vi "Read Input Registers1.vi"(7 "Unit_ID":T1={"Protocol ID"=0, "Unit ID"=1}, 8 "error in (no error)":errorcluster, 9 "number of input registers":u16, 10 "starting address":u16, 11 "Modbus master in":refnum<class "TCP.lvclass">) -> (0 "error out":errorcluster, 2 "register values":u16[](array[numeric]), 3 "Modbus master out":refnum<class "TCP.lvclass">)   [LabVIEW 2019, in "NI_modbus_upd.lvlib"]
doc: "Reads values from contiguous input registers. The maximum number of input registers this VI can read is 125."
uses:
  NI_modbus_upd.lvlib
  TCP/TCP.lvclass
  Ctl/Unit_ID.ctl
  TCP/TCP.lvclass/TCP.ctl
  Utility/Bytes to U16s1.vi
  Function code mismatch error1.vi
  Error Generator1.vi
  Read ADU Packet Master.vi
  Write ADU Packet Master.vi
  Modbus Data Unit (PDU)/Construct PDU1.vi
  Modbus Data Unit (PDU)/Unflatten to PDU1.vi
  TCP/Protocol Read.vi
  TCP/Protocol Write.vi
  <vilib>/Utility/error.llb/Error Cluster From Error Code.vi
  Modbus Data Unit (PDU)/Deconstruct PDU1.vi
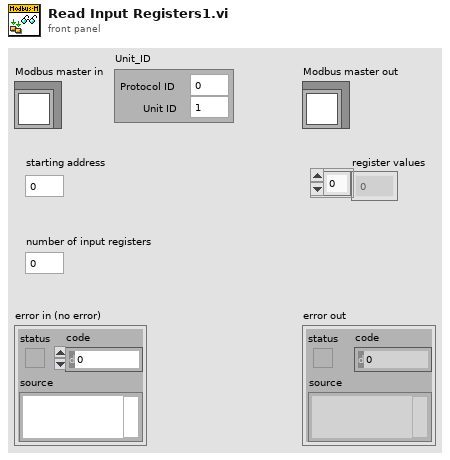
[diagram p1: front panel]
types:
  T1 = typedef "NI_modbus_upd.lvlib/Unit_ID.ctl" = cluster{"Protocol ID":u16, "Unit ID":u8}
  T2 = typedef "NI_modbus_upd.lvlib/MB Modbus Data Unit.ctl" = cluster{"function":T3, "Data":u8[]}
  T3 = typedef "NI_modbus_upd.lvlib/Function.ctl" = u8
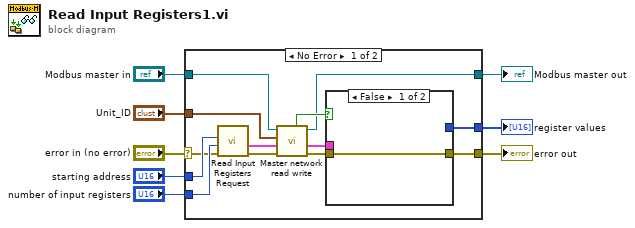
[diagram p0: block diagram]
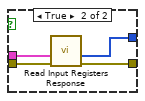
[diagram p2: hidden frame]
diagram:
  n1 = case shown="No Error" "error in (no error)" {
    selector: "error in (no error)" -> [w10 w28]
    tunnel: [w19 w28] -> w7
    tunnel: [w14 w27] -> w6
    tunnel: "Modbus master in" -> [w13 w27]
    tunnel: [w18 _] -> w4
    tunnel: "starting address" -> [w17 _]
    tunnel: "number of input registers" -> [w16 _]
    tunnel: "Unit_ID" -> [w11 _]
    frame No Error {
      n2 = call "Read Input Registers Request.vi"("error in (no error)"=w10, "number of registers"=w16, "starting address"=w17) -> ("error out"=w20:errorcluster, "Modbus Data Unit out"=w12:T2)  [unwired: 7 in]
      n3 = call "Master network read write.vi"("error in (no error)"=w20, "Modbus Data Unit"=w12, "Unit_ID"=w11, "TCP in"=w13) -> ("error out"=w21:errorcluster, "Modbus data unit out"=w9:T2, "TCP out"=w14:refnum<class "TCP.lvclass">, "PDU valid?"=w15:bool)  [unwired: 4 in]
      n4 = case shown="False" w15 {
        tunnel: w21 -> [w22 w26]
        tunnel: [w22 w25] -> w19
        tunnel: [_ w24] -> w18
        tunnel: w9 -> [_ w23]
        frame False {
        }
        frame True {
          n5 = call "Read Input Registers Response.vi"("error in (no error)"=w26, "Modbus Data Unit in"=w23) -> ("error out"=w25:errorcluster, "register values"=w24:u16[])  [unwired: 7 in, 1 out]
        }
      }
    }
    frame Error {
    }
  }
  "error out" <- w7
  "Modbus master out" <- w6
  "register values" <- w4
